vi "test Current Message Count.vi"(8 "error in (no error)":errorcluster, 11 "TestCase in":refnum<class "Message Queue Test Case.lvclass">) -> (0 "error out":errorcluster, 3 "TestCase out":refnum<class "Message Queue Test Case.lvclass">)   [LabVIEW 2017, in "Message Queue Test Case.lvclass"]
uses:
  Message Queue Test Case.lvclass
  Message Queue Test Case.lvclass/Message Queue Test Case.ctl
  Message/Abstract Message/Abstract Message.lvclass
  Message Queue/Abstract Message Queue/Abstract Message Queue.lvclass
  <vilib>/addons/_JKI Toolkits/VI Tester/TestCase.llb/TestCase.lvclass
  C:/Program Files (x86)/National Instruments/LabVIEW 2017/vi.lib/addons/_JKI Toolkits/VI Tester/TestCase.llb/TestCase.lvclass
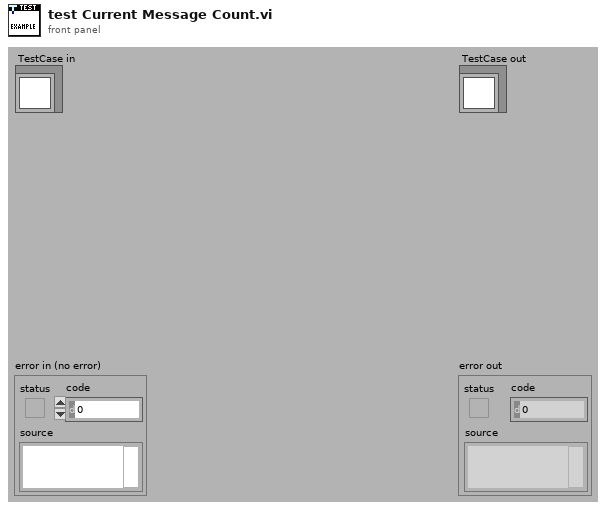
[diagram p1: front panel]
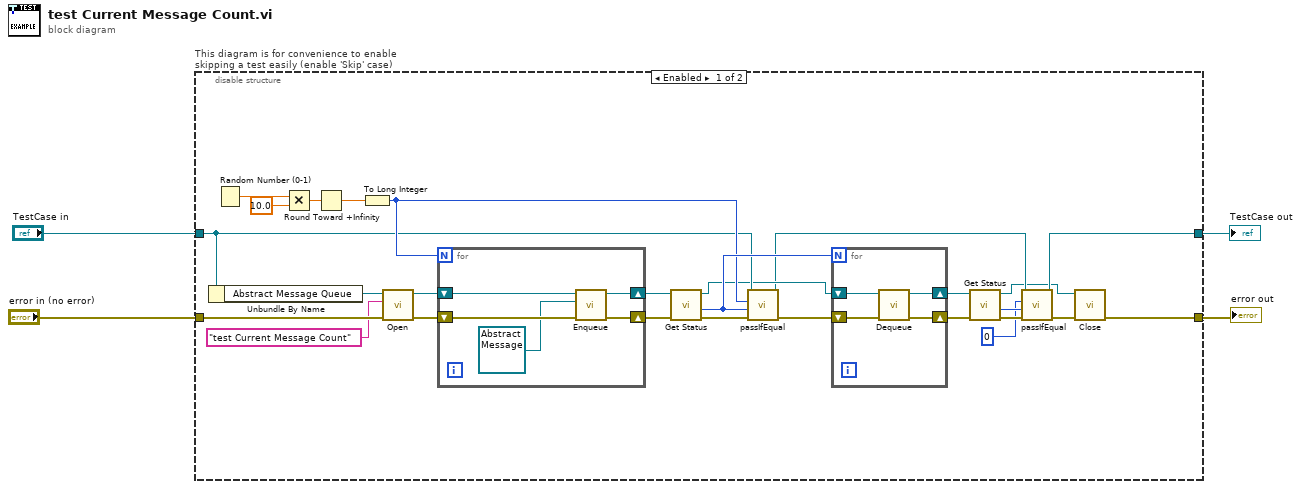
[diagram p0: block diagram]
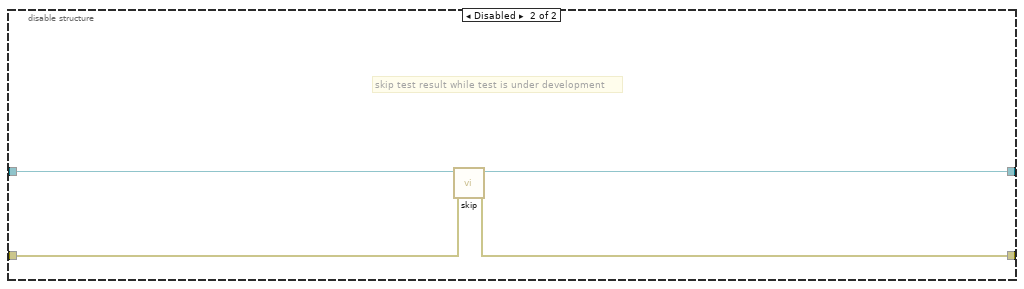
[diagram p2: hidden frame]
diagram:
  n1 = disable-structure "This diagram is for convenience to enable skipping a test easily (enable 'Skip' case)" shown="Enabled" {
    disable-tunnel: "TestCase in" -> [w14 w44]
    disable-tunnel: [w8 w42] -> w1
    disable-tunnel: [w6 w43] -> w3
    disable-tunnel: "error in (no error)" -> [w31 w41]
    frame Enabled {
      n2 = Unbundle By Name(w14) -> ("Abstract Message Queue"=w30:refnum<class "Abstract Message Queue.lvclass">)
      n3 = Random Number (0-1)() -> (number: 0 to 1=w28:dbl)
      n4 = Multiply(x=w28, y=10.0) -> (x*y=w26:dbl)
      n5 = Round Toward +Infinity(x=w26) -> (ceil(x): smallest int >= x=w21:dbl)
      n6 = To Long Integer(number=w21) -> (32bit integer=w15:i32)
      n7 = call-dynamic "Open.vi"("error in (no error)"=w31, "name (unnamed)"="test Current Message Count", "Abstract Message Queue in"=w30) -> ("error out"=w24:errorcluster, "Abstract Message Queue out"=w25:refnum<class "Abstract Message Queue.lvclass">)  [unwired: 7 in]
      n8 = for {
        N: w15 -> [_]
        shift-right: [w38] -> w22
        shift-left: w25 -> [w37]
        shift-right: [w39] -> w23
        shift-left: w24 -> [w40]
        n9 = call-dynamic "Enqueue.vi"("error in (no error)"=w40, "Message in"=refnum<class "Abstract Message.lvclass"> refnum, "Abstract Message Queue in"=w37) -> ("error out"=w39:errorcluster, "Abstract Message Queue out"=w38:refnum<class "Abstract Message Queue.lvclass">)  [unwired: 7 in]
      }
      n10 = call-dynamic "Get Status.vi"("error in (no error)"=w23, "Abstract Message Queue in"=w22) -> ("error out"=w20:errorcluster, "current number of messages"=w16:i32, "Abstract Message Queue out"=w13:refnum<class "Abstract Message Queue.lvclass">)  [unwired: 6 in, 1 out]
      n11 = call-dynamic "passIfEqual.vi"("error in (no error)"=w20, "y"=w16, "x"=w15, "TestCase in"=w14) -> ("error out"=w17:errorcluster, "TestCase out"=w9:refnum<class "Message Queue Test Case.lvclass">)  [unwired: 6 in]
      n12 = for {
        N: w16 -> [_]
        shift-right: [w33] -> w18
        shift-left: w13 -> [w34]
        shift-right: [w32] -> w19
        shift-left: w17 -> [w35]
        n13 = call-dynamic "Dequeue.vi"("error in (no error)"=w35, "Abstract Message Queue in"=w34) -> ("error out"=w32:errorcluster, "Abstract Message Queue out"=w33:refnum<class "Abstract Message Queue.lvclass">)  [unwired: 7 in, 1 out]
      }
      n14 = call-dynamic "Get Status.vi"("error in (no error)"=w19, "Abstract Message Queue in"=w18) -> ("error out"=w12:errorcluster, "current number of messages"=w11:i32, "Abstract Message Queue out"=w5:refnum<class "Abstract Message Queue.lvclass">)  [unwired: 6 in, 1 out]
      n15 = call-dynamic "passIfEqual.vi"("error in (no error)"=w12, "y"=w11, "x"=0 ("current number of messages"), "TestCase in"=w9) -> ("error out"=w7:errorcluster, "TestCase out"=w8:refnum<class "Message Queue Test Case.lvclass">)  [unwired: 6 in]
      n16 = call-dynamic "Close.vi"("error in (no error)"=w7, "Abstract Message Queue in"=w5) -> ("error out"=w6:errorcluster)  [unwired: 8 in, 1 out]
    }
    frame Disabled {
      # "skip test result while test is under development"
      n17 = call <vilib>:"skip.vi"("error in (no error)"=w41, "TestCase in"=w44) -> ("error out"=w43:errorcluster, "TestCase out"=w42:refnum<class "Message Queue Test Case.lvclass">)  [unwired: 8 in]
    }
  }
  "error out" <- w3
  "TestCase out" <- w1
